vi "get_attribute_int32_cmd_value.vi"(7 "Attribute":T1={"Identifier"="", "Descriptive Name"="", "Data Type"=enum."Integer 32", "Command"="", "Access"=enum."Read/Write", "Range Table"="", "Read Callback"="", "Write Callback"="", "Supported Models"="", "Instrument Options"="", "Index"=0, "OPC Wait"=FALSE, "No Status Check"=FALSE, "Cache Only"=FALSE}, 8 "error in":errorcluster caption="error in (no error)", 10 "Input Int32 value":i32, 11 "VISA resource name":refnum<visa-resource-name>) -> (0 "error out":errorcluster, 2 "Cmd Value out":string, 3 "VISA resource name out":refnum<visa-resource-name>)   [LabVIEW 2020, in "Rohde&Schwarz RTx Oscilloscopes.lvlib" / "rsidr_core.lvlib"]
doc: "Use this VI to covert the Int32 attribute value to the instrument command string when writing to the instrument.\nTakes the Int32 input value and converts it to the command string value.\nFor attributes with discrete range tables the value is converted to the corresponding enum string.\nOtherwise the VIs performs standard Int32->String conversion"
uses:
  rsidr_core.lvlib
  type_Attribute.ctl
  type_Attribute_Data_Type.ctl
  type_ReadWriteAccess.ctl
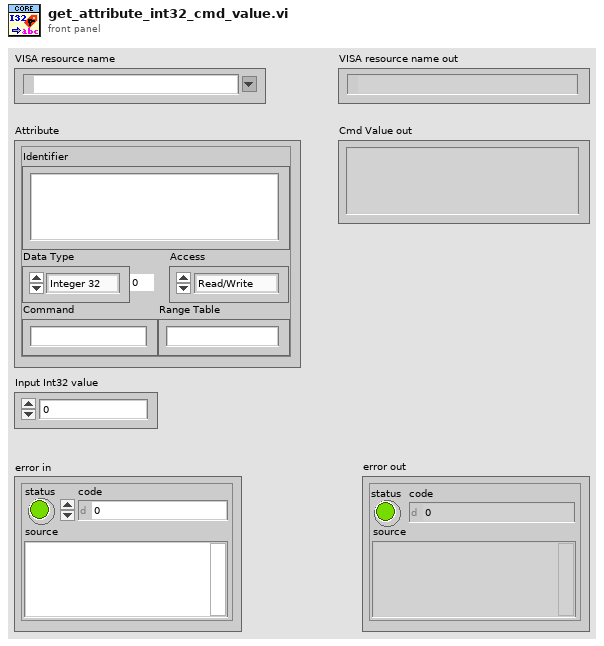
[diagram p1: front panel]
types:
  T1 = typedef "Rohde&Schwarz RTx Oscilloscopes.lvlib/rsidr_core.lvlib/type_Attribute.ctl" = cluster{"Identifier":string, "Descriptive Name":string, "Data Type":T2, "Command":string, "Access":T3, "Range Table":string, "Read Callback":string, "Write Callback":string, "Supported Models":string, "Instrument Options":string, "Index":i32, "OPC Wait":bool, "No Status Check":bool, "Cache Only":bool}
  T2 = typedef "Rohde&Schwarz RTx Oscilloscopes.lvlib/rsidr_core.lvlib/type_Attribute_Data_Type.ctl" = enum16{"Integer 32", "Double", "String", "Boolean", "None", "Integer 64", "RawString"}
  T3 = typedef "Rohde&Schwarz RTx Oscilloscopes.lvlib/rsidr_core.lvlib/type_ReadWriteAccess.ctl" = enum16{"Read Only", "Write Only", "Read/Write"}
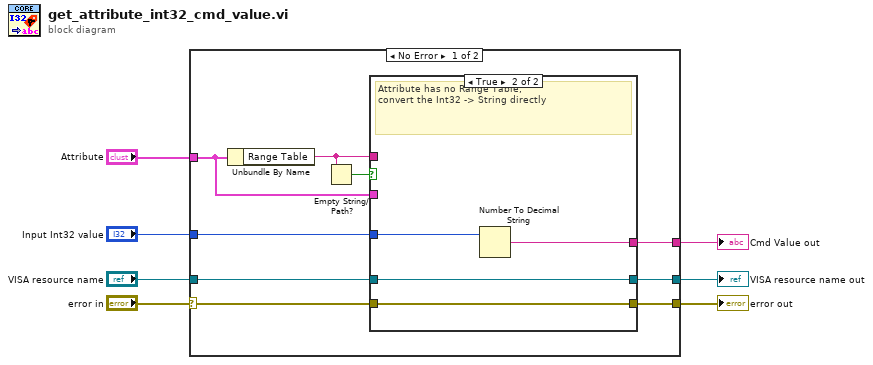
[diagram p0: block diagram]
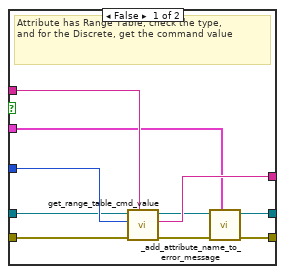
[diagram p2: hidden frame]
diagram:
  n1 = case shown="No Error" "error in" {
    selector: "error in" -> [w9 w32]
    tunnel: "VISA resource name" -> [w8 w31]
    tunnel: "Input Int32 value" -> [w16 _]
    tunnel: [w15 _] -> w6
    tunnel: [w14 w32] -> w5
    tunnel: [w13 w31] -> w4
    tunnel: "Attribute" -> [w10 _]
    frame No Error {
      n2 = Unbundle By Name(w10) -> ("Range Table"=w11:string)
      n3 = Empty String/Path?(string/path=w11) -> (empty?=w12:bool)
      n4 = case shown="True" w12 {
        tunnel: w9 -> [w18 w28]
        tunnel: w8 -> [w17 w27]
        tunnel: w16 -> [w26 w30]
        tunnel: [w24 w29] -> w15
        tunnel: [w21 w28] -> w14
        tunnel: [w20 w27] -> w13
        tunnel: w11 -> [w25 _]
        tunnel: w10 -> [w19 _]
        frame False {
          # "Attribute has Range Table, check the type,\nand for the Discrete, get the command value"
          n5 = call "get_range_table_cmd_value.vi"("Range Table ID in"=w25, "error in"=w18, "Input Int32 value"=w26, "VISA resource name"=w17) -> ("error out"=w23:errorcluster, "Cmd value out"=w24:string, "VISA resource name out"=w22:refnum<visa-resource-name>)  [unwired: 5 in]
          n6 = call "_add_attribute_name_to_error_message.vi"("Attribute"=w19, "error in"=w23, "VISA resource name"=w22) -> ("error out"=w21:errorcluster, "VISA resource name out"=w20:refnum<visa-resource-name>)  [unwired: 6 in, 1 out]
        }
        frame True {
          # "Attribute has no Range Table,\nconvert the Int32 -> String directly"
          n7 = Number To Decimal String(number=w30) -> (decimal integer string=w29:string)  [unwired: 1 in]
        }
      }
    }
    frame Error {
    }
  }
  "VISA resource name out" <- w4
  "error out" <- w5
  "Cmd Value out" <- w6
